vi "Graph.vi"(8 "error in (no error)":errorcluster, 9 "reset signal":bool, 11 "SignalIn.lvclass in":refnum<class "SignalIn.lvclass">) -> (0 "error out":errorcluster, 1 "signal out":waveform(dbl)(graph), 3 "SignalIn.lvclass out":refnum<class "SignalIn.lvclass">)   [LabVIEW 2011, in "SignalIn.lvclass"]
uses:
  SignalIn.lvclass
  SignalIn.lvclass/SignalIn.ctl
  <vilib>/measure/NI_MAPro.lvlib
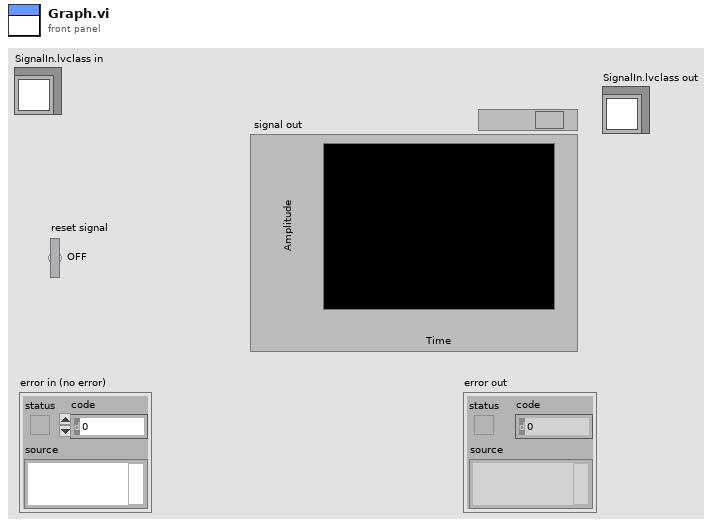
[diagram p1: front panel]
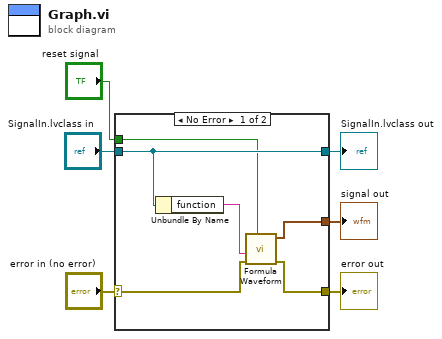
[diagram p0: block diagram]
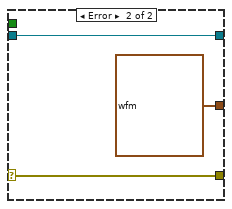
[diagram p2: hidden frame]
diagram:
  n1 = case shown="No Error" "error in (no error)" {
    selector: "error in (no error)" -> [w10 w15]
    tunnel: "SignalIn.lvclass in" -> [w12 w13]
    tunnel: "reset signal" -> [w8 _]
    tunnel: [w9 w15] -> w4
    tunnel: [w7 waveform(dbl) {"t0"=timestamp(0 s since 1904-01-01), "dt"=1.0, "Y"=[]} ("signal out")] -> w2
    tunnel: [w12 w13] -> w1
    frame No Error {
      n2 = Unbundle By Name(w12) -> ("function"=w11:string)
      n3 = call <vilib>:"Formula Waveform.vi"("reset signal"=w8, "error in (no error)"=w10, "formula"=w11) -> ("error out"=w9:errorcluster, "signal out"=w7:waveform(dbl))  [unwired: 7 in]
    }
    frame Error {
    }
  }
  "SignalIn.lvclass out" <- w1
  "error out" <- w4
  "signal out" <- w2
